vi "SP_OEE_2_test.vi"() -> ()   [LabVIEW 2017] (continued)
                      tunnel: [w13905] -> w13648
                      tunnel: w13663 -> [w13906]
                      tunnel: w13662 -> [w13902]
                      tunnel: [w13901] -> w13647
                      tunnel: w13661 -> [w13901]
                      tunnel: w13660 -> [w13962]
                      tunnel: w13659 -> [w13955]
                      tunnel: w13658 -> [w13946]
                      tunnel: w13657 -> [w13954]
                      tunnel: w13656 -> [w13944]
                      tunnel: w13655 -> [w13953]
                      tunnel: w13654 -> [w13942]
                      tunnel: w13653 -> [w13952]
                      tunnel: w13652 -> [w13940]
                      tunnel: w13651 -> [w13976]
                      tunnel: w13650 -> [w13975]
                      tunnel: w13649 -> [w13951]
                      tunnel: w13648 -> [w13938]
                      tunnel: [w13976] -> w13646
                      tunnel: [w13975] -> w13645
                      tunnel: [w13969] -> w13644
                      tunnel: [w13962] -> w13643
                      tunnel: [w13961] -> w13642
                      tunnel: [w13960] -> w13641
                      tunnel: [w13959] -> w13640
                      tunnel: [w13958] -> w13639
                      tunnel: [w13957] -> w13638
                      tunnel: [w13956] -> w13637
                      tunnel: [w13955] -> w13636
                      tunnel: [w13954] -> w13635
                      tunnel: [w13953] -> w13634
                      tunnel: [w13952] -> w13633
                      tunnel: [w13951] -> w13632
                      tunnel: [w13936] -> w13631
                      tunnel: w13647 -> [w13936]
                      tunnel: [w13989] -> _
                      tunnel: [w13985] -> _
                      tunnel: w13646 -> [w13986]
                      tunnel: w13645 -> [w13989]
                      tunnel: w13644 -> [w13980]
                      tunnel: w13643 -> [w13987]
                      tunnel: w13642 -> [_]
                      tunnel: w13641 -> [_]
                      tunnel: w13640 -> [w13977]
                      tunnel: w13639 -> [_]
                      tunnel: w13638 -> [_]
                      tunnel: w13637 -> [w13981]
                      tunnel: w13636 -> [_]
                      tunnel: w13635 -> [_]
                      tunnel: w13634 -> [w13978]
                      tunnel: w13633 -> [_]
                      tunnel: w13632 -> [_]
                      tunnel: w13631 -> [w13984]
                      frame #0 {
                        w13733 = "%Y-%m-%d" ("time format string (%c)")
                        n2498 = property on="Table" class="Tbl (strict)"("Visible"=TRUE) -> ()  [unwired: 2 in, 2 out]
                        n2499 = Format Date/Time String(time format string (%c)=w13733, seconds (now)=w13725) -> (date/time string=w13734:string)  [unwired: 1 in]
                        n2500 = Format Date/Time String(time format string (%c)=w13733, seconds (now)=w13724) -> (date/time string=w13732:string)  [unwired: 1 in]
                        n2501 = Format Into String(format string="Where BREAKDOWN_DATE between '%s' and '%s' ", w13734, w13732) -> (resulting string=w13731:string)  [unwired: 2 in, 1 out]
                        n2502 = call <vilib>:"DB Tools Select Data.vi"("condition"=w13731, "error in (no error)"=w13740, "columns"=string[] ["BREAKDOWN_DATE"], "table"="STATION_1_LOG_HISTORY", "connection reference"=w13742) -> ("error out"=w13727:errorcluster, "data"=w13730:variant[][], "connection reference out"=w13741:T2)  [unwired: 1 in]
                        n2503 = property on="Table 2" class="Tbl (strict)"("Visible"=FALSE) -> ()  [unwired: 2 in, 2 out]
                        n2504 = xnode "Database Variant To Data"("database variant"=w13730, "error in (no error)"=w13727, "type"=string[][] [] ("Elements Found")) -> ("data"=w13728:string[][], "error out"=w13726:errorcluster)
                        n2505 = Index Array(array=w13728, index (col)=0 ("disabled index (col)")) -> (element=w13736:string[])  [unwired: 1 in]
                        n2506 = call "Search_1d_array_element.vi"("Count in"=string[] [] ("Elements Found"), "BD Date"=w13736, "Elements Found in"=string[] [] ("Elements Found")) -> ("Elements Found out"=w13722:string[])  [unwired: 4 in, 2 out]
                        n2507 = Build Array(w13722) -> (w13746:string[][])
                        n2508 = Transpose 2D Array(2D array=w13746) -> (transposed array=w13745:string[][])
                      }
                      frame #1 {
                        n2509 = disable-structure shown="Enabled" {
                          disable-tunnel: w13806 -> [w13816 w13817]
                          disable-tunnel: [w13815 w13817] -> w13805
                          disable-tunnel: w13804 -> [w13814 w13818]
                          disable-tunnel: [w13813 w13818] -> w13803
                          disable-tunnel: w13801 -> [w13811 _]
                          disable-tunnel: w13800 -> [w13810 _]
                          disable-tunnel: [w13809 _] -> w13799
                          disable-tunnel: [w13808 _] -> w13796
                          disable-tunnel: w13794 -> [w13807 _]
                          frame Disabled {
                            n2510 = call "Stack_holderwise_total_bd_count_&_duration.vi"("Refnum in"=w13816, "BREAKDOWN_STK_HOLD_ID"=1, "condition"=w13807, "Form Date"=w13811, "To Date"=w13810, "error in (no error)"=w13814) -> ("Refnum out"=w13815:T2, "Count out"=w13809:string[], "appended array"=w13808:dbl[], "error out"=w13813:errorcluster)  [unwired: 6 in]
                          }
                          frame Enabled {
                          }
                        }
                        n2511 = call "NUMERIC TO STRING.vi"("appended array"=w13796) -> ("Array"=w13795:string[])  [unwired: 4 in]
                        n2512 = call "Insert_empty_element_with_zero.vi"("searched date"=w13799, "fixed date"=w13797) -> ("O/P"=w13792:string[])  [unwired: 9 in]
                        n2513 = call "Insert_empty_element_with_zero.vi"("searched date"=w13795, "fixed date"=w13797) -> ("O/P"=w13798:string[])  [unwired: 9 in]
                      }
                      frame #2 {
                        n2514 = disable-structure shown="Enabled" {
                          disable-tunnel: w13832 -> [w13845 w13847]
                          disable-tunnel: [w13844 w13847] -> w13831
                          disable-tunnel: w13830 -> [w13843 w13846]
                          disable-tunnel: [w13842 w13846] -> w13829
                          disable-tunnel: w13828 -> [w13841 _]
                          disable-tunnel: w13827 -> [w13840 _]
                          disable-tunnel: [w13839 _] -> w13826
                          disable-tunnel: [w13838 _] -> w13822
                          disable-tunnel: w13820 -> [w13837 _]
                          frame Disabled {
                            n2515 = call "Stack_holderwise_total_bd_count_&_duration.vi"("Refnum in"=w13843, "BREAKDOWN_STK_HOLD_ID"=2, "condition"=w13837, "Form Date"=w13841, "To Date"=w13840, "error in (no error)"=w13845) -> ("Refnum out"=w13842:T2, "Count out"=w13839:string[], "appended array"=w13838:dbl[], "error out"=w13844:errorcluster)  [unwired: 6 in]
                          }
                          frame Enabled {
                          }
                        }
                        n2516 = call "Insert_empty_element_with_zero.vi"("searched date"=w13826, "fixed date"=w13823) -> ("O/P"=w13825:string[])  [unwired: 9 in]
                        n2517 = call "NUMERIC TO STRING.vi"("appended array"=w13822) -> ("Array"=w13821:string[])  [unwired: 4 in]
                        n2518 = call "Insert_empty_element_with_zero.vi"("searched date"=w13821, "fixed date"=w13823) -> ("O/P"=w13824:string[])  [unwired: 9 in]
                      }
                      frame #3 {
                        n2519 = call "Stack_holderwise_total_bd_count_&_duration.vi"("Refnum in"=w13860, "BREAKDOWN_STK_HOLD_ID"=3, "condition"=w13850, "Form Date"=w13858, "To Date"=w13857, "error in (no error)"=w13862) -> ("Refnum out"=w13859:T2, "Count out"=w13856:string[], "appended array"=w13852:dbl[], "error out"=w13861:errorcluster)  [unwired: 6 in]
                        n2520 = call "Insert_empty_element_with_zero.vi"("searched date"=w13856, "fixed date"=w13853) -> ("O/P"=w13855:string[])  [unwired: 9 in]
                        n2521 = call "NUMERIC TO STRING.vi"("appended array"=w13852) -> ("Array"=w13851:string[])  [unwired: 4 in]
                        n2522 = call "Insert_empty_element_with_zero.vi"("searched date"=w13851, "fixed date"=w13853) -> ("O/P"=w13854:string[])  [unwired: 9 in]
                      }
                      frame #4 {
                        n2523 = disable-structure shown="Enabled" {
                          disable-tunnel: w13881 -> [w13897 w13900]
                          disable-tunnel: w13880 -> [w13896 w13899]
                          disable-tunnel: [w13895 w13899] -> w13879
                          disable-tunnel: [w13894 w13900] -> w13878
                          disable-tunnel: w13877 -> [w13893 _]
                          disable-tunnel: w13876 -> [w13892 _]
                          disable-tunnel: [w13891 _] -> w13875
                          disable-tunnel: [w13890 _] -> w13871
                          disable-tunnel: w13869 -> [w13889 _]
                          frame Disabled {
                            n2524 = call "Stack_holderwise_total_bd_count_&_duration.vi"("Refnum in"=w13896, "BREAKDOWN_STK_HOLD_ID"=4, "condition"=w13889, "Form Date"=w13893, "To Date"=w13892, "error in (no error)"=w13897) -> ("Refnum out"=w13895:T2, "Count out"=w13891:string[], "appended array"=w13890:dbl[], "error out"=w13894:errorcluster)  [unwired: 6 in]
                          }
                          frame Enabled {
                          }
                        }
                        n2525 = call "Insert_empty_element_with_zero.vi"("searched date"=w13875, "fixed date"=w13872) -> ("O/P"=w13874:string[])  [unwired: 9 in]
                        n2526 = call "NUMERIC TO STRING.vi"("appended array"=w13871) -> ("Array"=w13870:string[])  [unwired: 4 in]
                        n2527 = call "Insert_empty_element_with_zero.vi"("searched date"=w13870, "fixed date"=w13872) -> ("O/P"=w13873:string[])  [unwired: 9 in]
                      }
                      frame #5 {
                        n2528 = disable-structure shown="Enabled" {
                          disable-tunnel: w13914 -> [w13932 w13935]
                          disable-tunnel: [w13931 w13935] -> w13913
                          disable-tunnel: w13912 -> [w13930 w13934]
                          disable-tunnel: [w13929 w13934] -> w13911
                          disable-tunnel: w13910 -> [w13928 _]
                          disable-tunnel: w13909 -> [w13927 _]
                          disable-tunnel: [w13926 _] -> w13908
                          disable-tunnel: [w13925 _] -> w13904
                          disable-tunnel: w13902 -> [w13924 _]
                          frame Disabled {
                            n2529 = call "Stack_holderwise_total_bd_count_&_duration.vi"("Refnum in"=w13930, "BREAKDOWN_STK_HOLD_ID"=5, "condition"=w13924, "Form Date"=w13927, "To Date"=w13928, "error in (no error)"=w13932) -> ("Refnum out"=w13929:T2, "Count out"=w13926:string[], "appended array"=w13925:dbl[], "error out"=w13931:errorcluster)  [unwired: 6 in]
                          }
                          frame Enabled {
                          }
                        }
                        n2530 = call "NUMERIC TO STRING.vi"("appended array"=w13904) -> ("Array"=w13903:string[])  [unwired: 4 in]
                        n2531 = call "Insert_empty_element_with_zero.vi"("searched date"=w13908, "fixed date"=w13906) -> ("O/P"=w13907:string[])  [unwired: 9 in]
                        n2532 = call "Insert_empty_element_with_zero.vi"("searched date"=w13903, "fixed date"=w13906) -> ("O/P"=w13905:string[])  [unwired: 9 in]
                      }
                      frame #6 {
                        n2533 = call "String to numeric.vi"("Array"=w13946) -> ("Array 2"=w13945:dbl[])  [unwired: 4 in]
                        n2534 = call "String to numeric.vi"("Array"=w13944) -> ("Array 2"=w13943:dbl[])  [unwired: 4 in]
                        n2535 = call "String to numeric.vi"("Array"=w13942) -> ("Array 2"=w13941:dbl[])  [unwired: 4 in]
                        n2536 = call "String to numeric.vi"("Array"=w13940) -> ("Array 2"=w13939:dbl[])  [unwired: 4 in]
                        n2537 = call "String to numeric.vi"("Array"=w13938) -> ("Array 2"=w13937:dbl[])  [unwired: 4 in]
                        n2538 = Decimal String To Number(string=w13951) -> (number=w13970:i32[])  [unwired: 2 in, 1 out]
                        n2539 = Decimal String To Number(string=w13952) -> (number=w13971:i32[])  [unwired: 2 in, 1 out]
                        n2540 = Decimal String To Number(string=w13953) -> (number=w13972:i32[])  [unwired: 2 in, 1 out]
                        n2541 = Decimal String To Number(string=w13954) -> (number=w13973:i32[])  [unwired: 2 in, 1 out]
                        n2542 = Decimal String To Number(string=w13955) -> (number=w13968:i32[])  [unwired: 2 in, 1 out]
                        n2543 = Compound Arithmetic op=ADD(w13945, w13943, w13941, w13939, w13937) -> (w13948:dbl[])
                        n2544 = Build Array(w13946) -> (w13967:string[][])
                        n2545 = Build Array(w13944) -> (w13966:string[][])
                        n2546 = Build Array(w13942) -> (w13965:string[][])
                        n2547 = Build Array(w13940) -> (w13964:string[][])
                        n2548 = Build Array(w13938) -> (w13963:string[][])
                        n2549 = Number To Fractional String(number=w13948, precision (6)=i16 2) -> (F-format string=w13947:string[])  [unwired: 2 in]
                        n2550 = Compound Arithmetic op=ADD(w13970, w13971, w13972, w13973, w13968) -> (w13974:i32[])
                        n2551 = Transpose 2D Array(2D array=w13967) -> (transposed array=w13961:string[][])
                        n2552 = Transpose 2D Array(2D array=w13966) -> (transposed array=w13960:string[][])
                        n2553 = Transpose 2D Array(2D array=w13965) -> (transposed array=w13959:string[][])
                        n2554 = Transpose 2D Array(2D array=w13964) -> (transposed array=w13958:string[][])
                        n2555 = Transpose 2D Array(2D array=w13963) -> (transposed array=w13957:string[][])
                        n2556 = Number To Decimal String(number=w13974) -> (decimal integer string=w13969:string[])  [unwired: 1 in]
                        n2557 = Build Array(w13947) -> (w13950:string[][])
                        n2558 = Transpose 2D Array(2D array=w13950) -> (transposed array=w13956:string[][])
                      }
                      frame #7 {
                        w13979 = string[] [""]
                        n2559 = Insert Into Array(array=w13987, index (col)=1 ("disabled index (col)"), new element #1=w13979, new element #2=w13979, new element #3=w13979, new element #4=w13979, new element #5=w13978, new element #6=w13977, new element #7=w13979, new element #8=w13979, new element #9=w13979, new element #10=w13979, new element #11=w13980, new element #12=w13981) -> (w13983:string[][])  [unwired: 1 in]
                        n2560 = call "flot graph for month n year.vi"("BD Date"=w13984, "error in (no error)"=w13986, "Count total"=w13980) -> ("error out"=w13985:errorcluster, "Run-Time Status"=w13982:cluster{"Array 2":timestamp[], dbl[]})  [unwired: 7 in]
                        n2561 = local write "Run-Time Status"(w13982) -> ()
                        n2562 = local write "Table"(w13983) -> ()
                      }
                    }
                  }
                  frame "1" {
                    n2563 = flat-sequence {
                      tunnel: w13998 -> [w14112]
                      tunnel: w13997 -> [w14110]
                      tunnel: [w14096] -> w14088
                      tunnel: [w14111] -> w14087
                      tunnel: w13996 -> [_]
                      tunnel: [w14115] -> w14086
                      tunnel: [w14095] -> w14085
                      tunnel: [w14094] -> w14084
                      tunnel: [w14093] -> w14083
                      tunnel: w13995 -> [w14095]
                      tunnel: w13994 -> [w14094]
                      tunnel: ["Where BREAKDOWN_DATE between '%s'and '%s' and BREAKDOWN_STK_HOLD_ID ='%d' and  SHIFT_ID = '%d' "] -> w14082
                      tunnel: [w14093] -> w14081
                      tunnel: w13993 -> [w14089]
                      tunnel: [w14089] -> w13992
                      tunnel: w14088 -> [w14176]
                      tunnel: w14087 -> [w14178]
                      tunnel: w14086 -> [w14174]
                      tunnel: w14085 -> [w14173]
                      tunnel: w14084 -> [w14172]
                      tunnel: [w14175] -> w14080
                      tunnel: [w14177] -> w14079
                      tunnel: [w14174] -> w14078
                      tunnel: [w14164] -> w14077
                      tunnel: [w14170] -> w14076
                      tunnel: [w14173] -> w14075
                      tunnel: [w14172] -> w14074
                      tunnel: w14083 -> [w14169]
                      tunnel: [w14169] -> w14073
                      tunnel: w14082 -> [w14166]
                      tunnel: [w14166] -> w14072
                      tunnel: [w14165] -> w14071
                      tunnel: w14081 -> [w14165]
                      tunnel: w13992 -> [w14163]
                      tunnel: [w14162] -> w13991
                      tunnel: w14080 -> [w14208]
                      tunnel: w14079 -> [w14206]
                      tunnel: w14078 -> [w14211]
                      tunnel: w14077 -> [w14210]
                      tunnel: w14076 -> [w14209]
                      tunnel: w14075 -> [w14204]
                      tunnel: w14074 -> [w14203]
                      tunnel: [w14211] -> w14070
                      tunnel: [w14210] -> w14069
                      tunnel: [w14209] -> w14068
                      tunnel: [w14207] -> w14067
                      tunnel: [w14201] -> w14066
                      tunnel: [w14200] -> w14065
                      tunnel: [w14205] -> w14064
                      tunnel: [w14204] -> w14063
                      tunnel: [w14203] -> w14062
                      tunnel: w14073 -> [w14199]
                      tunnel: [w14199] -> w14061
                      tunnel: w14072 -> [w14196]
                      tunnel: [w14196] -> w14060
                      tunnel: [w14195] -> w14059
                      tunnel: w14071 -> [w14195]
                      tunnel: w13991 -> [w14194]
                      tunnel: [w14193] -> w13990
                      tunnel: w14070 -> [w14246]
                      tunnel: w14069 -> [w14245]
                      tunnel: w14068 -> [w14244]
                      tunnel: w14067 -> [w14241]
                      tunnel: w14066 -> [w14243]
                      tunnel: w14065 -> [w14242]
                      tunnel: w14064 -> [w14239]
                      tunnel: w14063 -> [w14237]
                      tunnel: w14062 -> [w14236]
                      tunnel: [w14246] -> w14058
                      tunnel: [w14245] -> w14057
                      tunnel: [w14244] -> w14056
                      tunnel: [w14243] -> w14055
                      tunnel: [w14242] -> w14054
                      tunnel: [w14240] -> w14053
                      tunnel: [w14234] -> w14052
                      tunnel: [w14233] -> w14051
                      tunnel: [w14238] -> w14050
                      tunnel: [w14237] -> w14049
                      tunnel: [w14236] -> w14048
                      tunnel: w14061 -> [w14232]
                      tunnel: [w14232] -> w14047
                      tunnel: w14060 -> [w14229]
                      tunnel: [w14229] -> w14046
                      tunnel: [w14228] -> w14045
                      tunnel: w14059 -> [w14228]
                      tunnel: w13990 -> [w14226]
                      tunnel: w14058 -> [w14267]
                      tunnel: w14057 -> [w14266]
                      tunnel: w14056 -> [w14265]
                      tunnel: w14055 -> [w14264]
                      tunnel: w14054 -> [w14263]
                      tunnel: w14053 -> [w14260]
                      tunnel: w14052 -> [w14262]
                      tunnel: w14051 -> [w14261]
                      tunnel: w14050 -> [w14259]
                      tunnel: w14049 -> [w14256]
                      tunnel: w14048 -> [w14255]
                      tunnel: [w14267] -> w14044
                      tunnel: [w14266] -> w14043
                      tunnel: [w14265] -> w14042
                      tunnel: [w14264] -> w14041
                      tunnel: [w14263] -> w14040
                      tunnel: [w14262] -> w14039
                      tunnel: [w14261] -> w14038
                      tunnel: [w14258] -> w14037
                      tunnel: [w14257] -> w14036
                      tunnel: [w14253] -> w14035
                      tunnel: [w14252] -> w14034
                      tunnel: [w14256] -> w14033
                      tunnel: [w14255] -> w14032
                      tunnel: w14047 -> [w14251]
                      tunnel: [w14251] -> w14031
                      tunnel: w14046 -> [w14248]
                      tunnel: [w14248] -> w14030
                      tunnel: [w14247] -> w14029
                      tunnel: w14045 -> [w14247]
                      tunnel: w14044 -> [w14302]
                      tunnel: w14043 -> [w14301]
                      tunnel: w14042 -> [w14300]
                      tunnel: w14041 -> [w14299]
                      tunnel: w14040 -> [w14298]
                      tunnel: w14039 -> [w14297]
                      tunnel: w14038 -> [w14296]
                      tunnel: w14037 -> [w14291]
                      tunnel: w14036 -> [w14293]
                      tunnel: w14035 -> [w14295]
                      tunnel: w14034 -> [w14294]
                      tunnel: w14033 -> [w14288]
                      tunnel: w14032 -> [w14289]
                      tunnel: [w14302] -> w14028
                      tunnel: [w14301] -> w14027
                      tunnel: [w14300] -> w14026
                      tunnel: [w14299] -> w14025
                      tunnel: [w14298] -> w14024
                      tunnel: [w14297] -> w14023
                      tunnel: [w14296] -> w14022
                      tunnel: [w14295] -> w14021
                      tunnel: [w14294] -> w14020
                      tunnel: [w14292] -> w14019
                      tunnel: [w14290] -> w14018
                      tunnel: [w14286] -> w14017
                      tunnel: [w14284] -> w14016
                      tunnel: w14031 -> [w14285]
                      tunnel: w14030 -> [w14281]
                      tunnel: [w14280] -> w14015
                      tunnel: w14029 -> [w14280]
                      tunnel: w14028 -> [w14341]
                      tunnel: w14027 -> [w14334]
                      tunnel: w14026 -> [w14325]
                      tunnel: w14025 -> [w14333]
                      tunnel: w14024 -> [w14323]
                      tunnel: w14023 -> [w14332]
                      tunnel: w14022 -> [w14321]
                      tunnel: w14021 -> [w14331]
                      tunnel: w14020 -> [w14319]
                      tunnel: w14019 -> [w14355]
                      tunnel: w14018 -> [w14354]
                      tunnel: w14017 -> [w14330]
                      tunnel: w14016 -> [w14317]
                      tunnel: [w14355] -> w14014
                      tunnel: [w14354] -> w14013
                      tunnel: [w14348] -> w14012
                      tunnel: [w14341] -> w14011
                      tunnel: [w14340] -> w14010
                      tunnel: [w14339] -> w14009
                      tunnel: [w14338] -> w14008
                      tunnel: [w14337] -> w14007
                      tunnel: [w14336] -> w14006
                      tunnel: [w14335] -> w14005
                      tunnel: [w14334] -> w14004
                      tunnel: [w14333] -> w14003
                      tunnel: [w14332] -> w14002
                      tunnel: [w14331] -> w14001
                      tunnel: [w14330] -> w14000
                      tunnel: [w14315] -> w13999
                      tunnel: w14015 -> [w14315]
                      tunnel: [w14368] -> _
                      tunnel: [w14364] -> _
                      tunnel: w14014 -> [w14365]
                      tunnel: w14013 -> [w14368]
                      tunnel: w14012 -> [w14359]
                      tunnel: w14011 -> [w14366]
                      tunnel: w14010 -> [_]
                      tunnel: w14009 -> [_]
                      tunnel: w14008 -> [w14358]
                      tunnel: w14007 -> [_]
                      tunnel: w14006 -> [_]
                      tunnel: w14005 -> [w14360]
                      tunnel: w14004 -> [_]
                      tunnel: w14003 -> [_]
                      tunnel: w14002 -> [w14356]
                      tunnel: w14001 -> [_]
                      tunnel: w14000 -> [_]
                      tunnel: w13999 -> [w14363]
                      frame #0 {
                        w14103 = "%Y-%m-%d" ("time format string (%c)")
                        n2564 = Decimal String To Number(string=w14089) -> (number=w14090:i32)  [unwired: 2 in, 1 out]
                        n2565 = property on="Table" class="Tbl (strict)"("Visible"=TRUE) -> ()  [unwired: 2 in, 2 out]
                        n2566 = Format Date/Time String(time format string (%c)=w14103, seconds (now)=w14095) -> (date/time string=w14104:string)  [unwired: 1 in]
                        n2567 = Format Date/Time String(time format string (%c)=w14103, seconds (now)=w14094) -> (date/time string=w14102:string)  [unwired: 1 in]
                        n2568 = Format Into String(format string="Where BREAKDOWN_DATE between '%s' and '%s' and  SHIFT_ID = '%d'  ", w14104, w14102, w14090) -> (resulting string=w14101:string)  [unwired: 2 in, 1 out]
                        n2569 = call <vilib>:"DB Tools Select Data.vi"("condition"=w14101, "error in (no error)"=w14110, "columns"=string[] ["BREAKDOWN_DATE"], "table"="STATION_1_LOG_HISTORY", "connection reference"=w14112) -> ("error out"=w14097:errorcluster, "data"=w14100:variant[][], "connection reference out"=w14111:T2)  [unwired: 1 in]
                        n2570 = property on="Table 2" class="Tbl (strict)"("Visible"=FALSE) -> ()  [unwired: 2 in, 2 out]
                        n2571 = xnode "Database Variant To Data"("database variant"=w14100, "error in (no error)"=w14097, "type"=string[][] [] ("Elements Found")) -> ("data"=w14098:string[][], "error out"=w14096:errorcluster)
                        n2572 = Index Array(array=w14098, index (col)=0 ("disabled index (col)")) -> (element=w14106:string[])  [unwired: 1 in]
                        n2573 = call "Search_1d_array_element.vi"("Count in"=string[] [] ("Elements Found"), "BD Date"=w14106, "Elements Found in"=string[] [] ("Elements Found")) -> ("Elements Found out"=w14093:string[])  [unwired: 4 in, 2 out]
                        n2574 = Build Array(w14093) -> (w14116:string[][])
                        n2575 = Transpose 2D Array(2D array=w14116) -> (transposed array=w14115:string[][])
                      }
                      frame #1 {
                        n2576 = disable-structure shown="Enabled" {
                          disable-tunnel: w14178 -> [w14189 w14191]
                          disable-tunnel: [w14188 w14191] -> w14177
                          disable-tunnel: w14176 -> [w14187 w14192]
                          disable-tunnel: [w14186 w14192] -> w14175
                          disable-tunnel: w14173 -> [w14184 _]
                          disable-tunnel: w14172 -> [w14183 _]
                          disable-tunnel: [w14182 _] -> w14171
                          disable-tunnel: [w14181 _] -> w14168
                          disable-tunnel: w14166 -> [w14180 _]
                          disable-tunnel: w14163 -> [w14179 w14190]
                          disable-tunnel: [_ w14190] -> w14162
                          frame Disabled {
                            n2577 = call "Stack_holderwise_total_bd_count_&_duration_2.vi"("Refnum in"=w14189, "BREAKDOWN_STK_HOLD_ID"=1, "condition"=w14180, "Form Date"=w14184, "To Date"=w14183, "error in (no error)"=w14187, "Shift"=w14179) -> ("Refnum out"=w14188:T2, "Count out"=w14182:string[], "appended array"=w14181:dbl[], "error out"=w14186:errorcluster)  [unwired: 5 in]
                          }
                          frame Enabled {
                          }
                        }
                        n2578 = call "NUMERIC TO STRING.vi"("appended array"=w14168) -> ("Array"=w14167:string[])  [unwired: 4 in]
                        n2579 = call "Insert_empty_element_with_zero.vi"("searched date"=w14171, "fixed date"=w14169) -> ("O/P"=w14164:string[])  [unwired: 9 in]
                        n2580 = call "Insert_empty_element_with_zero.vi"("searched date"=w14167, "fixed date"=w14169) -> ("O/P"=w14170:string[])  [unwired: 9 in]
                      }
                      frame #2 {
                        n2581 = disable-structure shown="Enabled" {
                          disable-tunnel: w14208 -> [w14222 w14224]
                          disable-tunnel: [w14221 w14224] -> w14207
                          disable-tunnel: w14206 -> [w14220 w14225]
                          disable-tunnel: [w14219 w14225] -> w14205
                          disable-tunnel: w14204 -> [w14218 _]
                          disable-tunnel: w14203 -> [w14217 _]
                          disable-tunnel: [w14216 _] -> w14202
                          disable-tunnel: [w14215 _] -> w14198
                          disable-tunnel: w14196 -> [w14214 _]
                          disable-tunnel: w14194 -> [w14212 w14223]
                          disable-tunnel: [_ w14223] -> w14193
                          frame Disabled {
                            n2582 = call "Stack_holderwise_total_bd_count_&_duration_2.vi"("Refnum in"=w14220, "BREAKDOWN_STK_HOLD_ID"=2, "condition"=w14214, "Form Date"=w14218, "To Date"=w14217, "error in (no error)"=w14222, "Shift"=w14212) -> ("Refnum out"=w14219:T2, "Count out"=w14216:string[], "appended array"=w14215:dbl[], "error out"=w14221:errorcluster)  [unwired: 5 in]
                          }
                          frame Enabled {
                          }
                        }
                        n2583 = call "Insert_empty_element_with_zero.vi"("searched date"=w14202, "fixed date"=w14199) -> ("O/P"=w14201:string[])  [unwired: 9 in]
                        n2584 = call "NUMERIC TO STRING.vi"("appended array"=w14198) -> ("Array"=w14197:string[])  [unwired: 4 in]
                        n2585 = call "Insert_empty_element_with_zero.vi"("searched date"=w14197, "fixed date"=w14199) -> ("O/P"=w14200:string[])  [unwired: 9 in]
                      }
                      frame #3 {
                        n2586 = call "Stack_holderwise_total_bd_count_&_duration_2.vi"("Refnum in"=w14239, "BREAKDOWN_STK_HOLD_ID"=3, "condition"=w14229, "Form Date"=w14237, "To Date"=w14236, "error in (no error)"=w14241, "Shift"=w14226) -> ("Refnum out"=w14238:T2, "Count out"=w14235:string[], "appended array"=w14231:dbl[], "error out"=w14240:errorcluster)  [unwired: 5 in]
                        n2587 = call "Insert_empty_element_with_zero.vi"("searched date"=w14235, "fixed date"=w14232) -> ("O/P"=w14234:string[])  [unwired: 9 in]
                        n2588 = call "NUMERIC TO STRING.vi"("appended array"=w14231) -> ("Array"=w14230:string[])  [unwired: 4 in]
                        n2589 = call "Insert_empty_element_with_zero.vi"("searched date"=w14230, "fixed date"=w14232) -> ("O/P"=w14233:string[])  [unwired: 9 in]
                      }
                      frame #4 {
                        n2590 = disable-structure shown="Enabled" {
                          disable-tunnel: w14260 -> [w14276 w14279]
                          disable-tunnel: w14259 -> [w14275 w14278]
                          disable-tunnel: [w14274 w14278] -> w14258
                          disable-tunnel: [w14273 w14279] -> w14257
                          disable-tunnel: w14256 -> [w14272 _]
                          disable-tunnel: w14255 -> [w14271 _]
                          disable-tunnel: [w14270 _] -> w14254
                          disable-tunnel: [w14269 _] -> w14250
                          disable-tunnel: w14248 -> [w14268 _]
                          frame Disabled {
                            n2591 = call "Stack_holderwise_total_bd_count_&_duration.vi"("Refnum in"=w14275, "BREAKDOWN_STK_HOLD_ID"=4, "condition"=w14268, "Form Date"=w14272, "To Date"=w14271, "error in (no error)"=w14276) -> ("Refnum out"=w14274:T2, "Count out"=w14270:string[], "appended array"=w14269:dbl[], "error out"=w14273:errorcluster)  [unwired: 6 in]
                          }
                          frame Enabled {
                          }
                        }
                        n2592 = call "Insert_empty_element_with_zero.vi"("searched date"=w14254, "fixed date"=w14251) -> ("O/P"=w14253:string[])  [unwired: 9 in]
                        n2593 = call "NUMERIC TO STRING.vi"("appended array"=w14250) -> ("Array"=w14249:string[])  [unwired: 4 in]
                        n2594 = call "Insert_empty_element_with_zero.vi"("searched date"=w14249, "fixed date"=w14251) -> ("O/P"=w14252:string[])  [unwired: 9 in]
                      }
                      frame #5 {
                        n2595 = disable-structure shown="Enabled" {
                          disable-tunnel: w14293 -> [w14311 w14314]
                          disable-tunnel: [w14310 w14314] -> w14292
                          disable-tunnel: w14291 -> [w14309 w14313]
                          disable-tunnel: [w14308 w14313] -> w14290
                          disable-tunnel: w14289 -> [w14307 _]
                          disable-tunnel: w14288 -> [w14306 _]
                          disable-tunnel: [w14305 _] -> w14287
                          disable-tunnel: [w14304 _] -> w14283
                          disable-tunnel: w14281 -> [w14303 _]
                          frame Disabled {
                            n2596 = call "Stack_holderwise_total_bd_count_&_duration.vi"("Refnum in"=w14309, "BREAKDOWN_STK_HOLD_ID"=5, "condition"=w14303, "Form Date"=w14306, "To Date"=w14307, "error in (no error)"=w14311) -> ("Refnum out"=w14308:T2, "Count out"=w14305:string[], "appended array"=w14304:dbl[], "error out"=w14310:errorcluster)  [unwired: 6 in]
                          }
                          frame Enabled {
                          }
                        }
                        n2597 = call "NUMERIC TO STRING.vi"("appended array"=w14283) -> ("Array"=w14282:string[])  [unwired: 4 in]
                        n2598 = call "Insert_empty_element_with_zero.vi"("searched date"=w14287, "fixed date"=w14285) -> ("O/P"=w14286:string[])  [unwired: 9 in]
                        n2599 = call "Insert_empty_element_with_zero.vi"("searched date"=w14282, "fixed date"=w14285) -> ("O/P"=w14284:string[])  [unwired: 9 in]
                      }
                      frame #6 {
                        n2600 = call "String to numeric.vi"("Array"=w14325) -> ("Array 2"=w14324:dbl[])  [unwired: 4 in]
                        n2601 = call "String to numeric.vi"("Array"=w14323) -> ("Array 2"=w14322:dbl[])  [unwired: 4 in]
                        n2602 = call "String to numeric.vi"("Array"=w14321) -> ("Array 2"=w14320:dbl[])  [unwired: 4 in]
                        n2603 = call "String to numeric.vi"("Array"=w14319) -> ("Array 2"=w14318:dbl[])  [unwired: 4 in]
                        n2604 = call "String to numeric.vi"("Array"=w14317) -> ("Array 2"=w14316:dbl[])  [unwired: 4 in]
                        n2605 = Decimal String To Number(string=w14330) -> (number=w14349:i32[])  [unwired: 2 in, 1 out]
                        n2606 = Decimal String To Number(string=w14331) -> (number=w14350:i32[])  [unwired: 2 in, 1 out]
                        n2607 = Decimal String To Number(string=w14332) -> (number=w14351:i32[])  [unwired: 2 in, 1 out]
                        n2608 = Decimal String To Number(string=w14333) -> (number=w14352:i32[])  [unwired: 2 in, 1 out]
                        n2609 = Decimal String To Number(string=w14334) -> (number=w14347:i32[])  [unwired: 2 in, 1 out]
                        n2610 = Compound Arithmetic op=ADD(w14324, w14322, w14320, w14318, w14316) -> (w14327:dbl[])
                        n2611 = Build Array(w14325) -> (w14346:string[][])
                        n2612 = Build Array(w14323) -> (w14345:string[][])
                        n2613 = Build Array(w14321) -> (w14344:string[][])
                        n2614 = Build Array(w14319) -> (w14343:string[][])
                        n2615 = Build Array(w14317) -> (w14342:string[][])
                        n2616 = Number To Fractional String(number=w14327, precision (6)=i16 2) -> (F-format string=w14326:string[])  [unwired: 2 in]
                        n2617 = Compound Arithmetic op=ADD(w14349, w14350, w14351, w14352, w14347) -> (w14353:i32[])
                        n2618 = Transpose 2D Array(2D array=w14346) -> (transposed array=w14340:string[][])
                        n2619 = Transpose 2D Array(2D array=w14345) -> (transposed array=w14339:string[][])
                        n2620 = Transpose 2D Array(2D array=w14344) -> (transposed array=w14338:string[][])
                        n2621 = Transpose 2D Array(2D array=w14343) -> (transposed array=w14337:string[][])
                        n2622 = Transpose 2D Array(2D array=w14342) -> (transposed array=w14336:string[][])
                        n2623 = Number To Decimal String(number=w14353) -> (decimal integer string=w14348:string[])  [unwired: 1 in]
                        n2624 = Build Array(w14326) -> (w14329:string[][])
                        n2625 = Transpose 2D Array(2D array=w14329) -> (transposed array=w14335:string[][])
                      }
                      frame #7 {
                        w14357 = string[] [""]
                        n2626 = Insert Into Array(array=w14366, index (col)=1 ("disabled index (col)"), new element #1=w14357, new element #2=w14357, new element #3=w14357, new element #4=w14357, new element #5=w14356, new element #6=w14358, new element #7=w14357, new element #8=w14357, new element #9=w14357, new element #10=w14357, new element #11=w14359, new element #12=w14360) -> (w14362:string[][])  [unwired: 1 in]
                        n2627 = call "flot graph for month n year.vi"("BD Date"=w14363, "error in (no error)"=w14365, "Count total"=w14359) -> ("error out"=w14364:errorcluster, "Run-Time Status"=w14361:cluster{"Array 2":timestamp[], dbl[]})  [unwired: 7 in]
                        n2628 = local write "Run-Time Status"(w14361) -> ()
                        n2629 = local write "Table"(w14362) -> ()
                      }
                    }
                  }
                  frame "2" {
                    n2630 = flat-sequence {
                      tunnel: w14377 -> [w14491]
                      tunnel: w14376 -> [w14489]
                      tunnel: [w14475] -> w14467
                      tunnel: [w14490] -> w14466
                      tunnel: w14375 -> [_]
                      tunnel: [w14494] -> w14465
                      tunnel: [w14474] -> w14464
                      tunnel: [w14473] -> w14463
                      tunnel: [w14472] -> w14462
                      tunnel: w14374 -> [w14474]
                      tunnel: w14373 -> [w14473]
                      tunnel: ["Where BREAKDOWN_DATE between '%s'and '%s' and BREAKDOWN_STK_HOLD_ID ='%d' and  SHIFT_ID = '%d' "] -> w14461
                      tunnel: [w14472] -> w14460
                      tunnel: w14372 -> [w14468]
                      tunnel: [w14468] -> w14371
                      tunnel: w14467 -> [w14555]
                      tunnel: w14466 -> [w14557]
                      tunnel: w14465 -> [w14553]
                      tunnel: w14464 -> [w14552]
                      tunnel: w14463 -> [w14551]
                      tunnel: [w14554] -> w14459
                      tunnel: [w14556] -> w14458
                      tunnel: [w14553] -> w14457
                      tunnel: [w14543] -> w14456
                      tunnel: [w14549] -> w14455
                      tunnel: [w14552] -> w14454
                      tunnel: [w14551] -> w14453
                      tunnel: w14462 -> [w14548]
                      tunnel: [w14548] -> w14452
                      tunnel: w14461 -> [w14545]
                      tunnel: [w14545] -> w14451
                      tunnel: [w14544] -> w14450
                      tunnel: w14460 -> [w14544]
                      tunnel: w14371 -> [w14542]
                      tunnel: [w14541] -> w14370
                      tunnel: w14459 -> [w14587]
                      tunnel: w14458 -> [w14585]
                      tunnel: w14457 -> [w14590]
                      tunnel: w14456 -> [w14589]
                      tunnel: w14455 -> [w14588]
                      tunnel: w14454 -> [w14583]
                      tunnel: w14453 -> [w14582]
                      tunnel: [w14590] -> w14449
                      tunnel: [w14589] -> w14448
                      tunnel: [w14588] -> w14447
                      tunnel: [w14586] -> w14446
                      tunnel: [w14580] -> w14445
                      tunnel: [w14579] -> w14444
                      tunnel: [w14584] -> w14443
                      tunnel: [w14583] -> w14442
                      tunnel: [w14582] -> w14441
                      tunnel: w14452 -> [w14578]
                      tunnel: [w14578] -> w14440
                      tunnel: w14451 -> [w14575]
                      tunnel: [w14575] -> w14439
                      tunnel: [w14574] -> w14438
                      tunnel: w14450 -> [w14574]
                      tunnel: w14370 -> [w14573]
                      tunnel: [w14572] -> w14369
                      tunnel: w14449 -> [w14625]
                      tunnel: w14448 -> [w14624]
                      tunnel: w14447 -> [w14623]
                      tunnel: w14446 -> [w14620]
                      tunnel: w14445 -> [w14622]
                      tunnel: w14444 -> [w14621]
                      tunnel: w14443 -> [w14618]
                      tunnel: w14442 -> [w14616]
                      tunnel: w14441 -> [w14615]
                      tunnel: [w14625] -> w14437
                      tunnel: [w14624] -> w14436
                      tunnel: [w14623] -> w14435
                      tunnel: [w14622] -> w14434
                      tunnel: [w14621] -> w14433
                      tunnel: [w14619] -> w14432
                      tunnel: [w14613] -> w14431
                      tunnel: [w14612] -> w14430
                      tunnel: [w14617] -> w14429
                      tunnel: [w14616] -> w14428
                      tunnel: [w14615] -> w14427
                      tunnel: w14440 -> [w14611]
                      tunnel: [w14611] -> w14426
                      tunnel: w14439 -> [w14608]
                      tunnel: [w14608] -> w14425
                      tunnel: [w14607] -> w14424
                      tunnel: w14438 -> [w14607]
                      tunnel: w14369 -> [w14605]
                      tunnel: w14437 -> [w14646]
                      tunnel: w14436 -> [w14645]
                      tunnel: w14435 -> [w14644]
                      tunnel: w14434 -> [w14643]
                      tunnel: w14433 -> [w14642]
                      tunnel: w14432 -> [w14639]
                      tunnel: w14431 -> [w14641]
                      tunnel: w14430 -> [w14640]
                      tunnel: w14429 -> [w14638]
                      tunnel: w14428 -> [w14635]
                      tunnel: w14427 -> [w14634]
                      tunnel: [w14646] -> w14423
                      tunnel: [w14645] -> w14422
                      tunnel: [w14644] -> w14421
                      tunnel: [w14643] -> w14420
                      tunnel: [w14642] -> w14419
                      tunnel: [w14641] -> w14418
                      tunnel: [w14640] -> w14417
                      tunnel: [w14637] -> w14416
                      tunnel: [w14636] -> w14415
                      tunnel: [w14632] -> w14414
                      tunnel: [w14631] -> w14413
                      tunnel: [w14635] -> w14412
                      tunnel: [w14634] -> w14411
                      tunnel: w14426 -> [w14630]
                      tunnel: [w14630] -> w14410
                      tunnel: w14425 -> [w14627]
                      tunnel: [w14627] -> w14409
                      tunnel: [w14626] -> w14408
                      tunnel: w14424 -> [w14626]
                      tunnel: w14423 -> [w14681]
                      tunnel: w14422 -> [w14680]
                      tunnel: w14421 -> [w14679]
                      tunnel: w14420 -> [w14678]
                      tunnel: w14419 -> [w14677]
                      tunnel: w14418 -> [w14676]
                      tunnel: w14417 -> [w14675]
                      tunnel: w14416 -> [w14670]
                      tunnel: w14415 -> [w14672]
                      tunnel: w14414 -> [w14674]
                      tunnel: w14413 -> [w14673]
                      tunnel: w14412 -> [w14667]
                      tunnel: w14411 -> [w14668]
                      tunnel: [w14681] -> w14407
                      tunnel: [w14680] -> w14406
                      tunnel: [w14679] -> w14405
                      tunnel: [w14678] -> w14404
                      tunnel: [w14677] -> w14403
                      tunnel: [w14676] -> w14402
                      tunnel: [w14675] -> w14401
                      tunnel: [w14674] -> w14400
                      tunnel: [w14673] -> w14399
                      tunnel: [w14671] -> w14398
                      tunnel: [w14669] -> w14397
                      tunnel: [w14665] -> w14396
                      tunnel: [w14663] -> w14395
                      tunnel: w14410 -> [w14664]
                      tunnel: w14409 -> [w14660]
                      tunnel: [w14659] -> w14394
                      tunnel: w14408 -> [w14659]
                      tunnel: w14407 -> [w14720]
                      tunnel: w14406 -> [w14713]
                      tunnel: w14405 -> [w14704]
                      tunnel: w14404 -> [w14712]
                      tunnel: w14403 -> [w14702]
                      tunnel: w14402 -> [w14711]
                      tunnel: w14401 -> [w14700]
                      tunnel: w14400 -> [w14710]
                      tunnel: w14399 -> [w14698]
                      tunnel: w14398 -> [w14734]
                      tunnel: w14397 -> [w14733]
                      tunnel: w14396 -> [w14709]
                      tunnel: w14395 -> [w14696]
                      tunnel: [w14734] -> w14393
                      tunnel: [w14733] -> w14392
                      tunnel: [w14727] -> w14391
                      tunnel: [w14720] -> w14390
                      tunnel: [w14719] -> w14389
                      tunnel: [w14718] -> w14388
                      tunnel: [w14717] -> w14387
                      tunnel: [w14716] -> w14386
                      tunnel: [w14715] -> w14385
                      tunnel: [w14714] -> w14384
                      tunnel: [w14713] -> w14383
                      tunnel: [w14712] -> w14382
                      tunnel: [w14711] -> w14381
                      tunnel: [w14710] -> w14380
                      tunnel: [w14709] -> w14379
                      tunnel: [w14694] -> w14378
                      tunnel: w14394 -> [w14694]
                      tunnel: [w14747] -> _
                      tunnel: [w14743] -> _
                      tunnel: w14393 -> [w14744]
                      tunnel: w14392 -> [w14747]
                      tunnel: w14391 -> [w14738]
                      tunnel: w14390 -> [w14745]
                      tunnel: w14389 -> [_]
                      tunnel: w14388 -> [_]
                      tunnel: w14387 -> [w14737]
                      tunnel: w14386 -> [_]
                      tunnel: w14385 -> [_]
                      tunnel: w14384 -> [w14739]
                      tunnel: w14383 -> [_]
                      tunnel: w14382 -> [_]
                      tunnel: w14381 -> [w14735]
                      tunnel: w14380 -> [_]
                      tunnel: w14379 -> [_]
                      tunnel: w14378 -> [w14742]
                      frame #0 {
                        w14482 = "%Y-%m-%d" ("time format string (%c)")
                        n2631 = Decimal String To Number(string=w14468) -> (number=w14469:i32)  [unwired: 2 in, 1 out]
                        n2632 = property on="Table" class="Tbl (strict)"("Visible"=TRUE) -> ()  [unwired: 2 in, 2 out]
                        n2633 = Format Date/Time String(time format string (%c)=w14482, seconds (now)=w14474) -> (date/time string=w14483:string)  [unwired: 1 in]
                        n2634 = Format Date/Time String(time format string (%c)=w14482, seconds (now)=w14473) -> (date/time string=w14481:string)  [unwired: 1 in]
                        n2635 = Format Into String(format string="Where BREAKDOWN_DATE between '%s' and '%s' and  SHIFT_ID = '%d'  ", w14483, w14481, w14469) -> (resulting string=w14480:string)  [unwired: 2 in, 1 out]
                        n2636 = call <vilib>:"DB Tools Select Data.vi"("condition"=w14480, "error in (no error)"=w14489, "columns"=string[] ["BREAKDOWN_DATE"], "table"="STATION_1_LOG_HISTORY", "connection reference"=w14491) -> ("error out"=w14476:errorcluster, "data"=w14479:variant[][], "connection reference out"=w14490:T2)  [unwired: 1 in]
                        n2637 = property on="Table 2" class="Tbl (strict)"("Visible"=FALSE) -> ()  [unwired: 2 in, 2 out]
                        n2638 = xnode "Database Variant To Data"("database variant"=w14479, "error in (no error)"=w14476, "type"=string[][] [] ("Elements Found")) -> ("data"=w14477:string[][], "error out"=w14475:errorcluster)
                        n2639 = Index Array(array=w14477, index (col)=0 ("disabled index (col)")) -> (element=w14485:string[])  [unwired: 1 in]
                        n2640 = call "Search_1d_array_element.vi"("Count in"=string[] [] ("Elements Found"), "BD Date"=w14485, "Elements Found in"=string[] [] ("Elements Found")) -> ("Elements Found out"=w14472:string[])  [unwired: 4 in, 2 out]
                        n2641 = Build Array(w14472) -> (w14495:string[][])
                        n2642 = Transpose 2D Array(2D array=w14495) -> (transposed array=w14494:string[][])
                      }
                      frame #1 {
                        n2643 = disable-structure shown="Enabled" {
                          disable-tunnel: w14557 -> [w14568 w14570]
                          disable-tunnel: [w14567 w14570] -> w14556
                          disable-tunnel: w14555 -> [w14566 w14571]
                          disable-tunnel: [w14565 w14571] -> w14554
                          disable-tunnel: w14552 -> [w14563 _]
                          disable-tunnel: w14551 -> [w14562 _]
                          disable-tunnel: [w14561 _] -> w14550
                          disable-tunnel: [w14560 _] -> w14547
                          disable-tunnel: w14545 -> [w14559 _]
                          disable-tunnel: w14542 -> [w14558 w14569]
                          disable-tunnel: [_ w14569] -> w14541
                          frame Disabled {
                            n2644 = call "Stack_holderwise_total_bd_count_&_duration_2.vi"("Refnum in"=w14568, "BREAKDOWN_STK_HOLD_ID"=1, "condition"=w14559, "Form Date"=w14563, "To Date"=w14562, "error in (no error)"=w14566, "Shift"=w14558) -> ("Refnum out"=w14567:T2, "Count out"=w14561:string[], "appended array"=w14560:dbl[], "error out"=w14565:errorcluster)  [unwired: 5 in]
                          }
                          frame Enabled {
                          }
                        }
                        n2645 = call "NUMERIC TO STRING.vi"("appended array"=w14547) -> ("Array"=w14546:string[])  [unwired: 4 in]
                        n2646 = call "Insert_empty_element_with_zero.vi"("searched date"=w14550, "fixed date"=w14548) -> ("O/P"=w14543:string[])  [unwired: 9 in]
                        n2647 = call "Insert_empty_element_with_zero.vi"("searched date"=w14546, "fixed date"=w14548) -> ("O/P"=w14549:string[])  [unwired: 9 in]
                      }
                      frame #2 {
                        n2648 = disable-structure shown="Enabled" {
                          disable-tunnel: w14587 -> [w14601 w14603]
                          disable-tunnel: [w14600 w14603] -> w14586
                          disable-tunnel: w14585 -> [w14599 w14604]
                          disable-tunnel: [w14598 w14604] -> w14584
                          disable-tunnel: w14583 -> [w14597 _]
                          disable-tunnel: w14582 -> [w14596 _]
                          disable-tunnel: [w14595 _] -> w14581
                          disable-tunnel: [w14594 _] -> w14577
                          disable-tunnel: w14575 -> [w14593 _]
                          disable-tunnel: w14573 -> [w14591 w14602]
                          disable-tunnel: [_ w14602] -> w14572
                          frame Disabled {
                            n2649 = call "Stack_holderwise_total_bd_count_&_duration_2.vi"("Refnum in"=w14599, "BREAKDOWN_STK_HOLD_ID"=2, "condition"=w14593, "Form Date"=w14597, "To Date"=w14596, "error in (no error)"=w14601, "Shift"=w14591) -> ("Refnum out"=w14598:T2, "Count out"=w14595:string[], "appended array"=w14594:dbl[], "error out"=w14600:errorcluster)  [unwired: 5 in]
                          }
                          frame Enabled {
                          }
                        }
                        n2650 = call "Insert_empty_element_with_zero.vi"("searched date"=w14581, "fixed date"=w14578) -> ("O/P"=w14580:string[])  [unwired: 9 in]
                        n2651 = call "NUMERIC TO STRING.vi"("appended array"=w14577) -> ("Array"=w14576:string[])  [unwired: 4 in]
                        n2652 = call "Insert_empty_element_with_zero.vi"("searched date"=w14576, "fixed date"=w14578) -> ("O/P"=w14579:string[])  [unwired: 9 in]
                      }
                      frame #3 {
                        n2653 = call "Stack_holderwise_total_bd_count_&_duration_2.vi"("Refnum in"=w14618, "BREAKDOWN_STK_HOLD_ID"=3, "condition"=w14608, "Form Date"=w14616, "To Date"=w14615, "error in (no error)"=w14620, "Shift"=w14605) -> ("Refnum out"=w14617:T2, "Count out"=w14614:string[], "appended array"=w14610:dbl[], "error out"=w14619:errorcluster)  [unwired: 5 in]
                        n2654 = call "Insert_empty_element_with_zero.vi"("searched date"=w14614, "fixed date"=w14611) -> ("O/P"=w14613:string[])  [unwired: 9 in]
                        n2655 = call "NUMERIC TO STRING.vi"("appended array"=w14610) -> ("Array"=w14609:string[])  [unwired: 4 in]
                        n2656 = call "Insert_empty_element_with_zero.vi"("searched date"=w14609, "fixed date"=w14611) -> ("O/P"=w14612:string[])  [unwired: 9 in]
                      }
                      frame #4 {
                        n2657 = disable-structure shown="Enabled" {
                          disable-tunnel: w14639 -> [w14655 w14658]
                          disable-tunnel: w14638 -> [w14654 w14657]
                          disable-tunnel: [w14653 w14657] -> w14637
                          disable-tunnel: [w14652 w14658] -> w14636
                          disable-tunnel: w14635 -> [w14651 _]
                          disable-tunnel: w14634 -> [w14650 _]
                          disable-tunnel: [w14649 _] -> w14633
                          disable-tunnel: [w14648 _] -> w14629
                          disable-tunnel: w14627 -> [w14647 _]
                          frame Disabled {
                            n2658 = call "Stack_holderwise_total_bd_count_&_duration.vi"("Refnum in"=w14654, "BREAKDOWN_STK_HOLD_ID"=4, "condition"=w14647, "Form Date"=w14651, "To Date"=w14650, "error in (no error)"=w14655) -> ("Refnum out"=w14653:T2, "Count out"=w14649:string[], "appended array"=w14648:dbl[], "error out"=w14652:errorcluster)  [unwired: 6 in]
                          }
                          frame Enabled {
                          }
                        }
                        n2659 = call "Insert_empty_element_with_zero.vi"("searched date"=w14633, "fixed date"=w14630) -> ("O/P"=w14632:string[])  [unwired: 9 in]
                        n2660 = call "NUMERIC TO STRING.vi"("appended array"=w14629) -> ("Array"=w14628:string[])  [unwired: 4 in]
                        n2661 = call "Insert_empty_element_with_zero.vi"("searched date"=w14628, "fixed date"=w14630) -> ("O/P"=w14631:string[])  [unwired: 9 in]
                      }
                      frame #5 {
                        n2662 = disable-structure shown="Enabled" {
                          disable-tunnel: w14672 -> [w14690 w14693]
                          disable-tunnel: [w14689 w14693] -> w14671
                          disable-tunnel: w14670 -> [w14688 w14692]
                          disable-tunnel: [w14687 w14692] -> w14669
                          disable-tunnel: w14668 -> [w14686 _]
                          disable-tunnel: w14667 -> [w14685 _]
                          disable-tunnel: [w14684 _] -> w14666
                          disable-tunnel: [w14683 _] -> w14662
                          disable-tunnel: w14660 -> [w14682 _]
                          frame Disabled {
                            n2663 = call "Stack_holderwise_total_bd_count_&_duration.vi"("Refnum in"=w14688, "BREAKDOWN_STK_HOLD_ID"=5, "condition"=w14682, "Form Date"=w14685, "To Date"=w14686, "error in (no error)"=w14690) -> ("Refnum out"=w14687:T2, "Count out"=w14684:string[], "appended array"=w14683:dbl[], "error out"=w14689:errorcluster)  [unwired: 6 in]
                          }
                          frame Enabled {
                          }
                        }
                        n2664 = call "NUMERIC TO STRING.vi"("appended array"=w14662) -> ("Array"=w14661:string[])  [unwired: 4 in]
                        n2665 = call "Insert_empty_element_with_zero.vi"("searched date"=w14666, "fixed date"=w14664) -> ("O/P"=w14665:string[])  [unwired: 9 in]
                        n2666 = call "Insert_empty_element_with_zero.vi"("searched date"=w14661, "fixed date"=w14664) -> ("O/P"=w14663:string[])  [unwired: 9 in]
                      }
                      frame #6 {
                        n2667 = call "String to numeric.vi"("Array"=w14704) -> ("Array 2"=w14703:dbl[])  [unwired: 4 in]
                        n2668 = call "String to numeric.vi"("Array"=w14702) -> ("Array 2"=w14701:dbl[])  [unwired: 4 in]
                        n2669 = call "String to numeric.vi"("Array"=w14700) -> ("Array 2"=w14699:dbl[])  [unwired: 4 in]
                        n2670 = call "String to numeric.vi"("Array"=w14698) -> ("Array 2"=w14697:dbl[])  [unwired: 4 in]
                        n2671 = call "String to numeric.vi"("Array"=w14696) -> ("Array 2"=w14695:dbl[])  [unwired: 4 in]
                        n2672 = Decimal String To Number(string=w14709) -> (number=w14728:i32[])  [unwired: 2 in, 1 out]
                        n2673 = Decimal String To Number(string=w14710) -> (number=w14729:i32[])  [unwired: 2 in, 1 out]
                        n2674 = Decimal String To Number(string=w14711) -> (number=w14730:i32[])  [unwired: 2 in, 1 out]
                        n2675 = Decimal String To Number(string=w14712) -> (number=w14731:i32[])  [unwired: 2 in, 1 out]
                        n2676 = Decimal String To Number(string=w14713) -> (number=w14726:i32[])  [unwired: 2 in, 1 out]
                        n2677 = Compound Arithmetic op=ADD(w14703, w14701, w14699, w14697, w14695) -> (w14706:dbl[])
                        n2678 = Build Array(w14704) -> (w14725:string[][])
                        n2679 = Build Array(w14702) -> (w14724:string[][])
                        n2680 = Build Array(w14700) -> (w14723:string[][])
                        n2681 = Build Array(w14698) -> (w14722:string[][])
                        n2682 = Build Array(w14696) -> (w14721:string[][])
                        n2683 = Number To Fractional String(number=w14706, precision (6)=i16 2) -> (F-format string=w14705:string[])  [unwired: 2 in]
                        n2684 = Compound Arithmetic op=ADD(w14728, w14729, w14730, w14731, w14726) -> (w14732:i32[])
                        n2685 = Transpose 2D Array(2D array=w14725) -> (transposed array=w14719:string[][])
                        n2686 = Transpose 2D Array(2D array=w14724) -> (transposed array=w14718:string[][])
                        n2687 = Transpose 2D Array(2D array=w14723) -> (transposed array=w14717:string[][])
                        n2688 = Transpose 2D Array(2D array=w14722) -> (transposed array=w14716:string[][])
                        n2689 = Transpose 2D Array(2D array=w14721) -> (transposed array=w14715:string[][])
                        n2690 = Number To Decimal String(number=w14732) -> (decimal integer string=w14727:string[])  [unwired: 1 in]
                        n2691 = Build Array(w14705) -> (w14708:string[][])
                        n2692 = Transpose 2D Array(2D array=w14708) -> (transposed array=w14714:string[][])
                      }
                      frame #7 {
                        w14736 = string[] [""]
                        n2693 = Insert Into Array(array=w14745, index (col)=1 ("disabled index (col)"), new element #1=w14736, new element #2=w14736, new element #3=w14736, new element #4=w14736, new element #5=w14735, new element #6=w14737, new element #7=w14736, new element #8=w14736, new element #9=w14736, new element #10=w14736, new element #11=w14738, new element #12=w14739) -> (w14741:string[][])  [unwired: 1 in]
                        n2694 = call "flot graph for month n year.vi"("BD Date"=w14742, "error in (no error)"=w14744, "Count total"=w14738) -> ("error out"=w14743:errorcluster, "Run-Time Status"=w14740:cluster{"Array 2":timestamp[], dbl[]})  [unwired: 7 in]
                        n2695 = local write "Run-Time Status"(w14740) -> ()
                        n2696 = local write "Table"(w14741) -> ()
                      }
                    }
                  }
                  frame "3" {
                    n2697 = flat-sequence {
                      tunnel: w14756 -> [w14870]
                      tunnel: w14755 -> [w14868]
                      tunnel: [w14854] -> w14846
                      tunnel: [w14869] -> w14845
                      tunnel: w14754 -> [_]
                      tunnel: [w14873] -> w14844
                      tunnel: [w14853] -> w14843
                      tunnel: [w14852] -> w14842
                      tunnel: [w14851] -> w14841
                      tunnel: w14753 -> [w14853]
                      tunnel: w14752 -> [w14852]
                      tunnel: ["Where BREAKDOWN_DATE between '%s'and '%s' and BREAKDOWN_STK_HOLD_ID ='%d' and  SHIFT_ID = '%d' "] -> w14840
                      tunnel: [w14851] -> w14839
                      tunnel: w14751 -> [w14847]
                      tunnel: [w14847] -> w14750
                      tunnel: w14846 -> [w14934]
                      tunnel: w14845 -> [w14936]
                      tunnel: w14844 -> [w14932]
                      tunnel: w14843 -> [w14931]
                      tunnel: w14842 -> [w14930]
                      tunnel: [w14933] -> w14838
                      tunnel: [w14935] -> w14837
                      tunnel: [w14932] -> w14836
                      tunnel: [w14922] -> w14835
                      tunnel: [w14928] -> w14834
                      tunnel: [w14931] -> w14833
                      tunnel: [w14930] -> w14832
                      tunnel: w14841 -> [w14927]
                      tunnel: [w14927] -> w14831
                      tunnel: w14840 -> [w14924]
                      tunnel: [w14924] -> w14830
                      tunnel: [w14923] -> w14829
                      tunnel: w14839 -> [w14923]
                      tunnel: w14750 -> [w14921]
                      tunnel: [w14920] -> w14749
                      tunnel: w14838 -> [w14966]
                      tunnel: w14837 -> [w14964]
                      tunnel: w14836 -> [w14969]
                      tunnel: w14835 -> [w14968]
                      tunnel: w14834 -> [w14967]
                      tunnel: w14833 -> [w14962]
                      tunnel: w14832 -> [w14961]
                      tunnel: [w14969] -> w14828
                      tunnel: [w14968] -> w14827
                      tunnel: [w14967] -> w14826
                      tunnel: [w14965] -> w14825
                      tunnel: [w14959] -> w14824
                      tunnel: [w14958] -> w14823
                      tunnel: [w14963] -> w14822
                      tunnel: [w14962] -> w14821
                      tunnel: [w14961] -> w14820
                      tunnel: w14831 -> [w14957]
                      tunnel: [w14957] -> w14819
                      tunnel: w14830 -> [w14954]
                      tunnel: [w14954] -> w14818
                      tunnel: [w14953] -> w14817
                      tunnel: w14829 -> [w14953]
                      tunnel: w14749 -> [w14952]
                      tunnel: [w14951] -> w14748
                      tunnel: w14828 -> [w15004]
                      tunnel: w14827 -> [w15003]
                      tunnel: w14826 -> [w15002]
                      tunnel: w14825 -> [w14999]
                      tunnel: w14824 -> [w15001]
                      tunnel: w14823 -> [w15000]
                      tunnel: w14822 -> [w14997]
                      tunnel: w14821 -> [w14995]
                      tunnel: w14820 -> [w14994]
                      tunnel: [w15004] -> w14816
                      tunnel: [w15003] -> w14815
                      tunnel: [w15002] -> w14814
                      tunnel: [w15001] -> w14813
                      tunnel: [w15000] -> w14812
                      tunnel: [w14998] -> w14811
                      tunnel: [w14992] -> w14810
                      tunnel: [w14991] -> w14809
                      tunnel: [w14996] -> w14808
                      tunnel: [w14995] -> w14807
                      tunnel: [w14994] -> w14806
                      tunnel: w14819 -> [w14990]
                      tunnel: [w14990] -> w14805
                      tunnel: w14818 -> [w14987]
                      tunnel: [w14987] -> w14804
                      tunnel: [w14986] -> w14803
                      tunnel: w14817 -> [w14986]
                      tunnel: w14748 -> [w14984]
                      tunnel: w14816 -> [w15025]
                      tunnel: w14815 -> [w15024]
                      tunnel: w14814 -> [w15023]
                      tunnel: w14813 -> [w15022]
                      tunnel: w14812 -> [w15021]
                      tunnel: w14811 -> [w15018]
                      tunnel: w14810 -> [w15020]
                      tunnel: w14809 -> [w15019]
                      tunnel: w14808 -> [w15017]
                      tunnel: w14807 -> [w15014]
                      tunnel: w14806 -> [w15013]
                      tunnel: [w15025] -> w14802
                      tunnel: [w15024] -> w14801
                      tunnel: [w15023] -> w14800
                      tunnel: [w15022] -> w14799
                      tunnel: [w15021] -> w14798
                      tunnel: [w15020] -> w14797
                      tunnel: [w15019] -> w14796
                      tunnel: [w15016] -> w14795
                      tunnel: [w15015] -> w14794
                      tunnel: [w15011] -> w14793
                      tunnel: [w15010] -> w14792
                      tunnel: [w15014] -> w14791
                      tunnel: [w15013] -> w14790
                      tunnel: w14805 -> [w15009]
                      tunnel: [w15009] -> w14789
                      tunnel: w14804 -> [w15006]
                      tunnel: [w15006] -> w14788
                      tunnel: [w15005] -> w14787
                      tunnel: w14803 -> [w15005]
                      tunnel: w14802 -> [w15060]
                      tunnel: w14801 -> [w15059]
                      tunnel: w14800 -> [w15058]
                      tunnel: w14799 -> [w15057]
                      tunnel: w14798 -> [w15056]
                      tunnel: w14797 -> [w15055]
                      tunnel: w14796 -> [w15054]
                      tunnel: w14795 -> [w15049]
                      tunnel: w14794 -> [w15051]
                      tunnel: w14793 -> [w15053]
                      tunnel: w14792 -> [w15052]
                      tunnel: w14791 -> [w15046]
                      tunnel: w14790 -> [w15047]
                      tunnel: [w15060] -> w14786
                      tunnel: [w15059] -> w14785
                      tunnel: [w15058] -> w14784
                      tunnel: [w15057] -> w14783
                      tunnel: [w15056] -> w14782
                      tunnel: [w15055] -> w14781
                      tunnel: [w15054] -> w14780
                      tunnel: [w15053] -> w14779
                      tunnel: [w15052] -> w14778
                      tunnel: [w15050] -> w14777
                      tunnel: [w15048] -> w14776
                      tunnel: [w15044] -> w14775
                      tunnel: [w15042] -> w14774
                      tunnel: w14789 -> [w15043]
                      tunnel: w14788 -> [w15039]
                      tunnel: [w15038] -> w14773
                      tunnel: w14787 -> [w15038]
                      tunnel: w14786 -> [w15099]
                      tunnel: w14785 -> [w15092]
